vi "Save As Measurement Service template.vi"(8 "error in":errorcluster, 10 "Measurement Service Name":string, 11 "Project ref":refnum<vi>) -> (0 "error out":errorcluster)   [LabVIEW 2020, in "MeasurementService Editor.lvlib"]
uses:
  MeasurementService Editor.lvlib
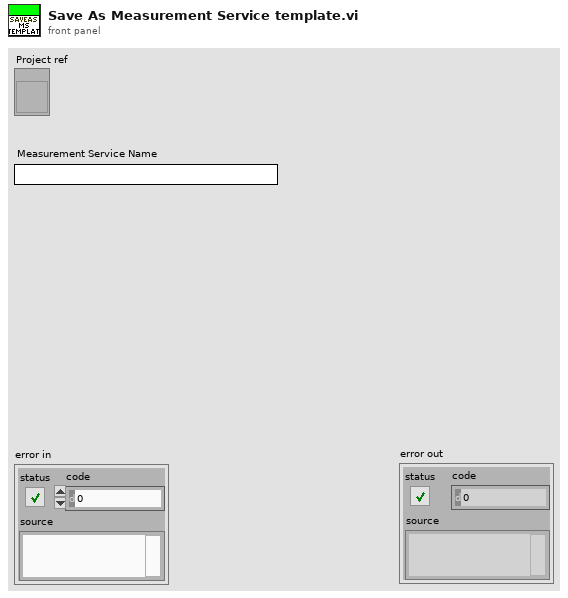
[diagram p1: front panel]
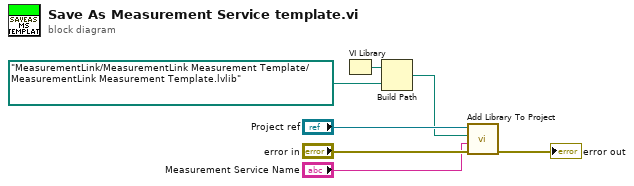
[diagram p0: block diagram]
diagram:
  n1 = VI Library() -> (path=w3:path)
  n2 = Build Path(base path=w3, name or relative path=path "MeasurementLink/MeasurementLink Measurement Template/MeasurementLink Measurement Template.lvlib" ("Library Path")) -> (appended path=w1:path)
  n3 = call "Add Library To Project.vi"("error in"="error in", "New Library Name"="Measurement Service Name", "Library Path"=w1, "Project ref"="Project ref") -> ("error out"=→"error out":errorcluster)  [unwired: 7 in]
